vi "Show Front Panel.vi"(8 "error in (no error)":errorcluster, 11 "JQMHCore in":refnum<class "RQMHModule.lvclass">) -> (0 "error out":errorcluster, 3 "JQMHCore out":refnum<class "RQMHModule.lvclass">)   [LabVIEW 2024, in "RQMHModule.lvclass"]
uses:
  RQMHModule.lvclass
  Show Front Panel--Args.ctl
  RQMHModule.lvclass/RQMHModule.ctl
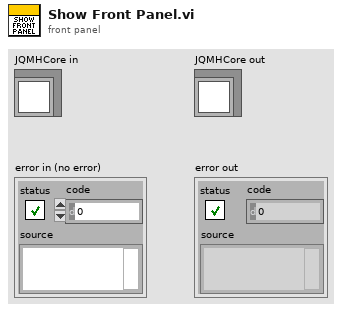
[diagram p1: front panel]
types:
  T1 = typedef "RQMHModule.lvclass/Show Front Panel--Args.ctl" = variant
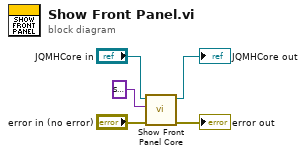
[diagram p0: block diagram]
diagram:
  n1 = call "Show Front Panel Core.vi"("error in (no error)"="error in (no error)", "Data"=T1 variant, "JQMHCore in"="JQMHCore in") -> ("error out"=→"error out":errorcluster, "JQMHCore out"=→"JQMHCore out":refnum<class "RQMHModule.lvclass">)  [unwired: 7 in]
